vi "ref.vi"() -> ()   [LabVIEW 2020]
uses:
  <vilib>/Utility/traverseref.llb/TRef TravTarget.ctl
  <vilib>/Utility/traverseref.llb/VI Scripting - Traverse.lvlib
panel:
  out "只遍历循环 2":string[][](table) caption="只遍历循环"
  in  "Path to target VI":path=path "Test - Using Traverse.vi"
  out "所有对象[]":string[][](table)
  out "只遍历循环":string[][](table)
  out "遍历全部":string[][](table)
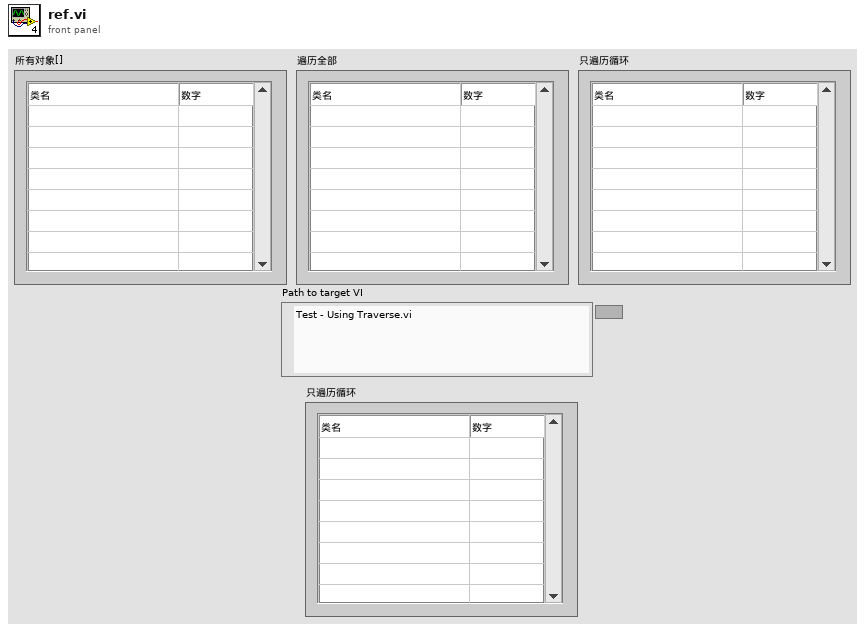
[diagram p1: front panel]
types:
  T1 = typedef "TRef TravTarget.ctl" = enum16{"FP", "BD", "Other"}
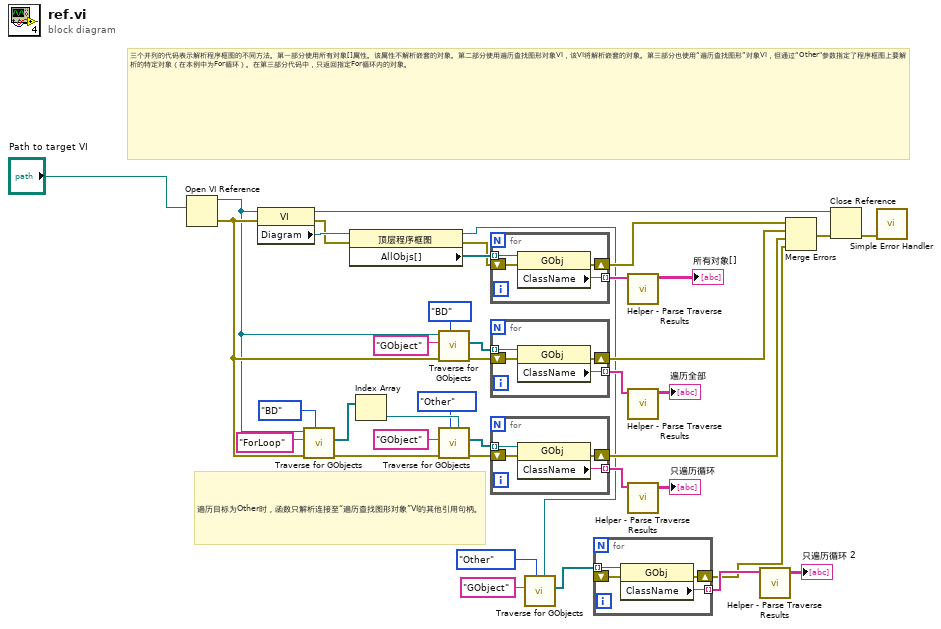
[diagram p0: block diagram]
diagram:
  # "遍历目标为Other时，函数只解析连接至“遍历查找图形对象”VI的其他引用句柄。"
  # "三个并列的代码表示解析程序框图的不同方法。第一部分使用所有对象[]属性。该属性不解析嵌套的对象。第二部分使用遍历查找图形对象VI，该VI将解析嵌套的对象。第三部分也使用“遍历查找图形”对象VI，但通过“Other\"参数指定了程序框图上要解析的特定对象（在本例中为For循环）。在第三部分代码中，只返回指定For循环内的对象。"
  n1 = Open VI Reference(vi path="Path to target VI") -> (vi reference=w29:refnum<vi>, error out=w30:errorcluster)  [unwired: 5 in]
  n2 = property class="VI"(reference=w29, error in=w30) -> (reference out=w36:refnum<vi>, error out=w26:errorcluster, "Diagram"=w27:refnum<vi>)
  n3 = call <vilib>:"Traverse for GObjects.vi"("Traverse Target"=TRef_TravTarget."BD", "error in (no error)"=w30, "Class Name"="ForLoop", "VI Refnum"=w29) -> ("error out"=w32:errorcluster, "References"=w33:refnum<vi>[])  [unwired: 4 in, 2 out]
  n4 = property class="顶层程序框图"(reference=w27, error in=w26) -> (reference out=w3:refnum<vi>, error out=w25:errorcluster, "AllObjs[]"=w28:refnum<vi>[])
  n5 = Index Array(array=w33) -> (element=w34:refnum<vi>)  [unwired: 1 in]
  n6 = call <vilib>:"Traverse for GObjects.vi"("Traverse Target"=TRef_TravTarget."BD", "error in (no error)"=w30, "Class Name"="GObject", "VI Refnum"=w29) -> ("error out"=w18:errorcluster, "References"=w19:refnum<vi>[])  [unwired: 4 in, 2 out]
  n7 = call <vilib>:"Traverse for GObjects.vi"("Other Refnum"=w34, "Traverse Target"=TRef_TravTarget."Other", "error in (no error)"=w32, "Class Name"="GObject") -> ("error out"=w11:errorcluster, "References"=w10:refnum<vi>[])  [unwired: 4 in, 2 out]
  n8 = for {
    tunnel: w28 -> [w43] mode=indexing
    tunnel: [w42] -> w23 mode=indexing
    shift-right: [w40] -> w37
    shift-left: w25 -> [w41]
    n9 = property class="GObj"(reference=w43, error in=w41) -> (error out=w40:errorcluster, "ClassName"=w42:string)  [unwired: 1 out]
  }
  n10 = for {
    tunnel: w19 -> [w47] mode=indexing
    tunnel: [w46] -> w16 mode=indexing
    shift-right: [w44] -> w17
    shift-left: w18 -> [w45]
    n11 = property class="GObj"(reference=w47, error in=w45) -> (error out=w44:errorcluster, "ClassName"=w46:string)  [unwired: 1 out]
  }
  n12 = for {
    tunnel: w10 -> [w51] mode=indexing
    tunnel: [w50] -> w8 mode=indexing
    shift-right: [w48] -> w9
    shift-left: w11 -> [w49]
    n13 = property class="GObj"(reference=w51, error in=w49) -> (error out=w48:errorcluster, "ClassName"=w50:string)  [unwired: 1 out]
  }
  n14 = call <vilib>:"Traverse for GObjects.vi"("Other Refnum"=w3, "Traverse Target"=TRef_TravTarget."Other", "Class Name"="GObject") -> ("References"=w7:refnum<vi>[])  [unwired: 5 in, 3 out]
  n15 = for {
    tunnel: w7 -> [w55] mode=indexing
    tunnel: [w54] -> w5 mode=indexing
    shift-right: [w52] -> w4
    shift-left: _ -> [w53]
    n16 = property class="GObj"(reference=w55, error in=w53) -> (error out=w52:errorcluster, "ClassName"=w54:string)  [unwired: 1 out]
  }
  n17 = call "Helper - Parse Traverse Results.vi"("遍历结果"=w23) -> ("解析结果"=→"所有对象[]":string[][])  [unwired: 10 in]
  n18 = call "Helper - Parse Traverse Results.vi"("遍历结果"=w16) -> ("解析结果"=→"遍历全部":string[][])  [unwired: 10 in]
  n19 = call "Helper - Parse Traverse Results.vi"("遍历结果"=w8) -> ("解析结果"=→"只遍历循环":string[][])  [unwired: 10 in]
  n20 = call "Helper - Parse Traverse Results.vi"("遍历结果"=w5) -> ("解析结果"=→"只遍历循环 2":string[][])  [unwired: 10 in]
  n21 = Merge Errors(w37, w17, w9, w4) -> (w24:errorcluster)
  n22 = Close Reference(reference=w36, error in (no error)=w24) -> (error out=w38:errorcluster)
  n23 = call <vilib>:"Simple Error Handler.vi"("error in (no error)"=w38) -> ()  [unwired: 4 in, 5 out]
